vi "Create Arbitrary Waveform [ARB] Core.vi"(8 "error in (no error)":errorcluster, 9 "waveform data array (empty)":dbl[](array[numeric]) format="%.3f", 11 "IVI_Fgen in":refnum<class "IVI_Fgen.lvclass">) -> (0 "error out":errorcluster, 2 "waveform handle":i32, 3 "IVI_Fgen out":refnum<class "IVI_Fgen.lvclass">)   [LabVIEW 2013, in "IVI_Fgen.lvlib" / "IVI_Fgen.lvclass"]
doc: "This VI creates an arbitrary waveform and returns a handle that identifies that waveform. You pass this handle to the IviFgen Configure Arbitrary Waveform [ARB] VI to produce that waveform. You also use the handles this VI returns to specify a sequence of arbitrary waveforms with the IviFgen Create Arbitrary Sequence [SEQ] VI.\n\nNotes:\n\n(1) This VI is part of the IviFgenArbWfm [ARB] extension group."
uses:
  IVI_Fgen.lvclass
  IVI_Fgen.lvclass/IVI_Fgen.ctl
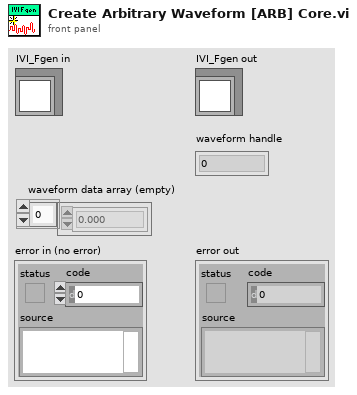
[diagram p1: front panel]
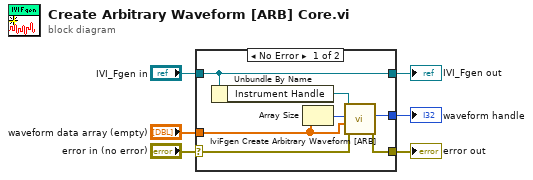
[diagram p0: block diagram]
diagram:
  n1 = case shown="No Error" "error in (no error)" {
    selector: "error in (no error)" -> [w11 w15]
    tunnel: [w10 w15] -> w5
    tunnel: [w13 w14] -> w3
    tunnel: "IVI_Fgen in" -> [w13 w14]
    tunnel: "waveform data array (empty)" -> [w7 _]
    tunnel: [w9 _] -> w1
    frame No Error {
      n2 = Unbundle By Name(w13) -> ("Instrument Handle"=w12:refnum<k15>)
      n3 = Array Size(array=w7) -> (size(s)=w8:i32)
      n4 = call <vilib>:"IviFgen Create Arbitrary Waveform [ARB].vi"("error in (no error)"=w11, "waveform data array (empty)"=w7, "waveform size (0)"=w8, "instrument handle"=w12) -> ("error out"=w10:errorcluster, "waveform handle"=w9:i32)  [unwired: 5 in, 1 out]
    }
    frame Error {
    }
  }
  "error out" <- w5
  "IVI_Fgen out" <- w3
  "waveform handle" <- w1
